vi "Update.vi"(8 "error in (no error)":errorcluster, 11 "PongSwitch in":refnum<class "SnakeSwitch.lvclass">) -> (0 "error out":errorcluster, 3 "PongSwitch out":refnum<class "SnakeSwitch.lvclass">)   [LabVIEW 2019]
uses:
  SnakeSwitch.lvclass
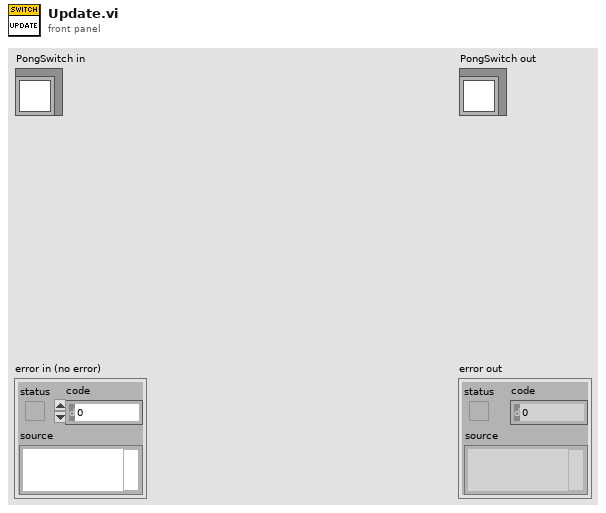
[diagram p1: front panel]
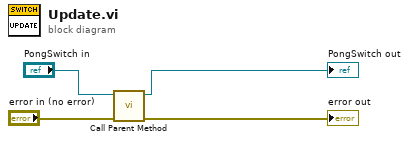
[diagram p0: block diagram]
diagram:
  n1 = call-parent "Call Parent Method"("error in (no error)"="error in (no error)", "GameObject in"="PongSwitch in") -> ("error out"=→"error out":errorcluster, "GameObject out"=→"PongSwitch out":refnum<class "SnakeSwitch.lvclass">)  [unwired: 8 in]
